vi "visn_Calculate CRC-16 (Bits Array)Fer.vi"(11 "Bits Array":u8[](array[numeric])=[1, 1, 0, 0, 1, 1, 1, 0, 1, 0] format="%0x") -> (3 "CRC-16":u8[](array[numeric])=[1, 0, 0, 0, 0, 0, 0, 0, 0, 0, 0, 0, 0, 0, 0, 0] format="%0x")   [LabVIEW 2015]
panel:
  out "hex crc16":string[](array[string])
  out "bool":bool[](array[boolean])
  out "loop":i32
  # "1"
  # "2"
  # "3"
  # "4"
  # "5"
  # "6"
  # "7"
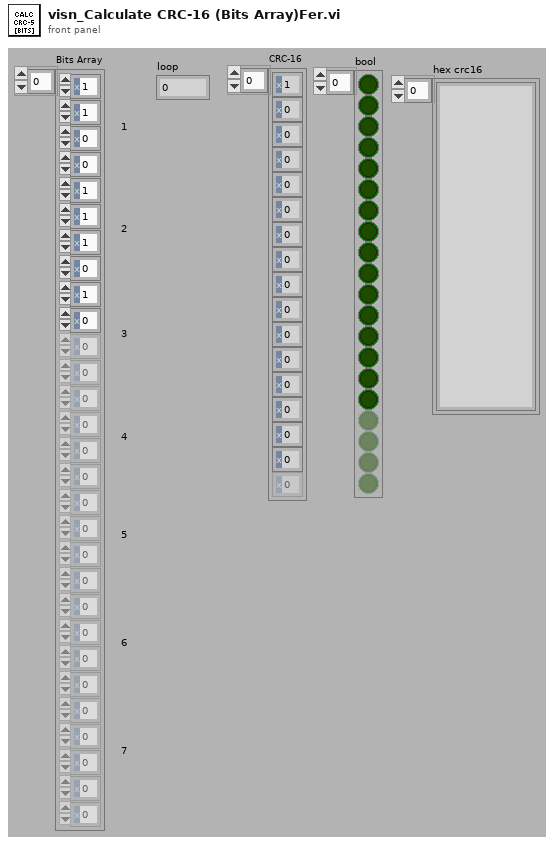
[diagram p1: front panel]
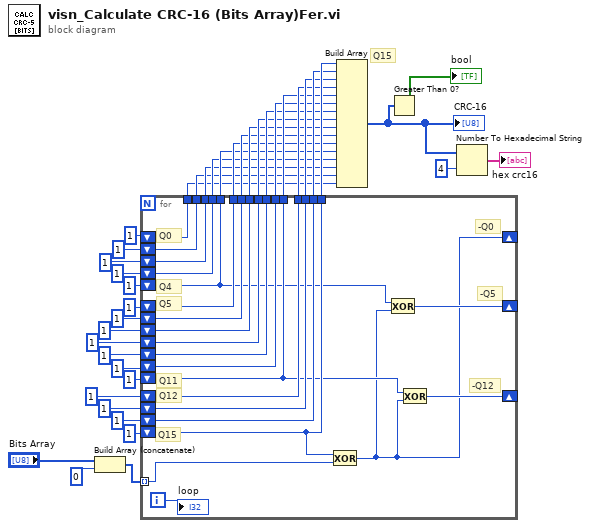
[diagram p0: block diagram]
diagram:
  # "Q15"
  n1 = Build Array (concatenate)("Bits Array", u8 0) -> (w39:u8[])
  n2 = for {
    tunnel: w39 -> [w45] mode=indexing
    shift-right: [w42] -> _
    shift-left: u8 1 -> [w55]
    shift-left: u8 1 -> [w54]
    shift-left: u8 1 -> [w53]
    shift-right: [w44] -> _
    shift-left: u8 1 -> [w49]
    shift-left: u8 1 -> [w48]
    shift-left: u8 1 -> [w47]
    shift-left: u8 1 -> [w46]
    shift-left: u8 1 -> [w52]
    shift-left: u8 1 -> [w51]
    shift-left: u8 1 -> [w50]
    shift-left: u8 1 -> [w43]
    shift-right: [w41] -> _
    shift-left: u8 1 -> [w59]
    shift-left: u8 1 -> [w58]
    shift-left: u8 1 -> [w57]
    shift-left: u8 1 -> [w56]
    shift-left: u8 1 -> [w40]
    tunnel: [w59] -> w5
    tunnel: [w58] -> w6
    tunnel: [w57] -> w7
    tunnel: [w56] -> w8
    tunnel: [w40] -> w9
    tunnel: [w55] -> w10
    tunnel: [w54] -> w11
    tunnel: [w53] -> w12
    tunnel: [w52] -> w13
    tunnel: [w51] -> w14
    tunnel: [w50] -> w15
    tunnel: [w43] -> w16
    tunnel: [w49] -> w17
    tunnel: [w48] -> w18
    tunnel: [w47] -> w19
    tunnel: [w46] -> w20
    i -> [w60]
    # "Q12"
    # "Q5"
    # "Q0"
    # "-Q12"
    # "-Q5"
    # "-Q0"
    # "Q4"
    # "Q11"
    # "-Q12"
    # "-Q0"
    # "-Q5"
    # "Q15"
    n3 = Exclusive Or(1:w45, 2:w46) -> (0:w41:u8)
    n4 = Exclusive Or(1:w41, 2:w40) -> (0:w42:u8)
    n5 = Exclusive Or(1:w41, 2:w43) -> (0:w44:u8)
    "loop" <- w60
  }
  n6 = Build Array(w20, w19, w18, w17, w16, w15, w14, w13, w12, w11, w10, w9, w8, w7, w6, w5) -> (w3:u8[])
  "CRC-16" <- w3
  n7 = Greater Than 0?(x=w3) -> (x > 0?=→"bool":bool[])
  n8 = Number To Hexadecimal String(1:i16 4 ("width (-)"), 2:w3) -> (0:→"hex crc16":string[])
